vi "Y Cluster Values.vi"(11 "Clust Refnum":refnum<vi>) -> (3 "Array":sgl[](array[numeric]))   [LabVIEW 2016, in "M1M3SupportEUI_Views.lvlib"]
uses:
  M1M3SupportEUI_Views.lvlib
panel:
  # "Y"
  # "0"
  # "1"
  # "2"
  # "3"
  # "4"
  # "5"
  # "6"
  # "7"
  # "8"
  # "9"
  # "100"
  # "110"
  # "120"
  # "130"
  # "200"
  # "210"
  # "220"
  # "230"
  # "300"
  # "310"
  # "320"
  # "330"
  # "400"
  # "410"
  # "420"
  # "430"
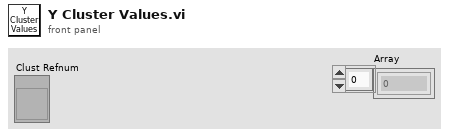
[diagram p1: front panel]
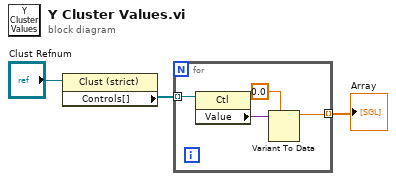
[diagram p0: block diagram]
diagram:
  n1 = property on="Property Node" class="Clust (strict)"(reference="Clust Refnum") -> ("Controls[]"=w3:refnum<vi>[])  [unwired: 1 in, 2 out]
  n2 = for {
    tunnel: w3 -> [w7] mode=indexing
    tunnel: [w4] -> w1 mode=indexing
    n3 = property on="Property Node" class="Ctl"(reference=w7) -> ("Value"=w6:variant)  [unwired: 1 in, 2 out]
    n4 = Variant To Data(type=sgl 0.0, Variant=w6) -> (data=w4:sgl)  [unwired: 1 in, 1 out]
  }
  "Array" <- w1
